vi "Main.vi"(11 "Module Admin":refnum<class "Delacor_lib_QMH_Module Admin.lvclass">) -> ()   [LabVIEW 2021, in "Safety & Release Configuration.lvlib"]
doc: "This template is based off of the Queued Message Handler design pattern and the Queued Message Handler project template that ships with LabVIEW.\n\nThe main difference is that the queue is private to this module and communication between modules is performed via Broadcast and Request events.\n\nRequest events are wrapped in public API methods and are handled in the Event Handling Loop (EHL) of this VI. Any module can register for Broadcast events sent by this module. The EHL generates messages based on user interface actions.\n\nThe Message Handling Loop (MHL) processes messages generated by the EHL, or by other messages. The messages are string values, so new messages can be added easily to the Message Cases case structure in the MHL. Each message cluster can also provide an optional value for Message Data, which is a variant that can be converted to whatever message-specific data is required.\n_____\nBased on DQMH Project Template 7.0.1.1316."
uses:
  Safety & Release Configuration.lvlib
  <vilib>/Delacor/Delacor QMH/Libraries/Module Admin_class/Delacor_lib_QMH_Module Admin.lvclass
  Module Data--cluster.ctl
  Do Something Argument--cluster.ctl
  <vilib>/Delacor/Delacor QMH/Libraries/Message Queue_class/Delacor_lib_QMH_Message Queue.lvclass/Delacor_lib_QMH_Message Queue.ctl
  Do Something Else Argument--cluster.ctl
  Do Something Else and Wait for Reply Argument--cluster.ctl
  Do Something Else and Wait (Reply Payload)--cluster.ctl
  Stop Argument--cluster.ctl
  <vilib>/Delacor/Delacor QMH/Libraries/Module Admin_class/Delacor_lib_QMH_Module Admin.lvclass/Delacor_lib_QMH_Module Admin.ctl
  <vilib>/Utility/miscctls.llb/LVPointTypeDef.ctl
  <vilib>/Delacor/Delacor QMH/Libraries/Message Queue_class/Delacor_lib_QMH_Enqueue Message (Single).vi
  <vilib>/Delacor/Delacor QMH/Libraries/Module Admin_class/Delacor_lib_QMH_Get External Launch.vi
  <vilib>/Delacor/Delacor QMH/Libraries/Message Queue_class/Delacor_lib_QMH_Message Queue.lvclass
  <userlib>/_OpenG.lib/appcontrol/appcontrol.llb/openg_application_control.lvlib
panel:
  in  "Main Tab":enum32{"Release Module", "Safety Module"}(tab)
  in  "Release Module Tab":T1(tab)
  in  "Proximity Sensor 2":u16(ring) items=["Release_Module/port0/line0", "Release_Module/port0/line1", "Release_Module/port0/line2", "Release_Module/port0/line3", "Release_Module/port0/line4", "Release_Module/port0/line5", "Release_Module/port0/line6", "Release_Module/port0/line7", "Release_Module/port0/line8", "Release_Module/port0/line9", "Release_Module/port0/line10", "Release_Module/port0/line11", "Release_Module/port0/line12", "Release_Module/port0/line13", "Release_Module/port0/line14", "Release_Module/port0/line15"]
  in  "Proximity sensor 1":u16(ring) items=["Release_Module/port0/line0", "Release_Module/port0/line1", "Release_Module/port0/line2", "Release_Module/port0/line3", "Release_Module/port0/line4", "Release_Module/port0/line5", "Release_Module/port0/line6", "Release_Module/port0/line7", "Release_Module/port0/line8", "Release_Module/port0/line9", "Release_Module/port0/line10", "Release_Module/port0/line11", "Release_Module/port0/line12", "Release_Module/port0/line13", "Release_Module/port0/line14", "Release_Module/port0/line15"]
  in  "Solenoid Valve":u16(ring) items=["Release_Module/port1/line0", "Release_Module/port1/line1", "Release_Module/port1/line2", "Release_Module/port1/line3", "Release_Module/port1/line4", "Release_Module/port1/line5", "Release_Module/port1/line6", "Release_Module/port1/line7", "Release_Module/port1/line8", "Release_Module/port1/line9", "Release_Module/port1/line10", "Release_Module/port1/line11", "Release_Module/port1/line12", "Release_Module/port1/line13", "Release_Module/port1/line14", "Release_Module/port1/line15"]
  in  "Safety Module Tab":T1(tab)
  in  "Safety Sensor 3":u16(ring) items=["Saftey_Module/port0/line0", "Saftey_Module/port0/line1", "Saftey_Module/port0/line2", "Saftey_Module/port0/line3"]
  in  "Safety Sensor 2":u16(ring) items=["Saftey_Module/port0/line0", "Saftey_Module/port0/line1", "Saftey_Module/port0/line2", "Saftey_Module/port0/line3"]
  in  "Safety Sensor 1":u16(ring) items=["Saftey_Module/port0/line0", "Saftey_Module/port0/line1", "Saftey_Module/port0/line2", "Saftey_Module/port0/line3"]
  in  "Safety Valve 3":u16(ring) items=["Saftey_Module/port0/line4", "Saftey_Module/port0/line5", "Saftey_Module/port0/line6", "Saftey_Module/port0/line7"]
  in  "Safety Valve 2":u16(ring) items=["Saftey_Module/port0/line4", "Saftey_Module/port0/line5", "Saftey_Module/port0/line6", "Saftey_Module/port0/line7"]
  in  "Safety Valve 1":u16(ring) items=["Saftey_Module/port0/line4", "Saftey_Module/port0/line5", "Saftey_Module/port0/line6", "Saftey_Module/port0/line7"]
  in  "Save":bool
  in  "Exit":bool
  out "error out":errorcluster
  out "X":dbl
  out "Status":string
  in  "Simulate MHL Error":bool
  in  "Simulate EHL Error":bool
  in  "Do Something Else <Replace Me>":bool
  in  "Do Something <Replace Me>":bool
  # "IIT-M Drop Tower Test System"
  # "Safety & Release Configuration Window"
  # "These controls have associated \"Value Changed\" events configured in the Event Structure on the diagram.\n\nReplace them (and reconfigure the Event Structure) with the controls you need for your application. \n\nOther processes communicate with this Module via its Public API (wrappers for its Request Events).\n\nThis Module communicates with other processes via its Broadcast Events.\nAny process that wants to receive these messages can register for this module's Broadcast events."
  # "This template is for the DQMH framework. See the block diagram for more information on how to use this template."
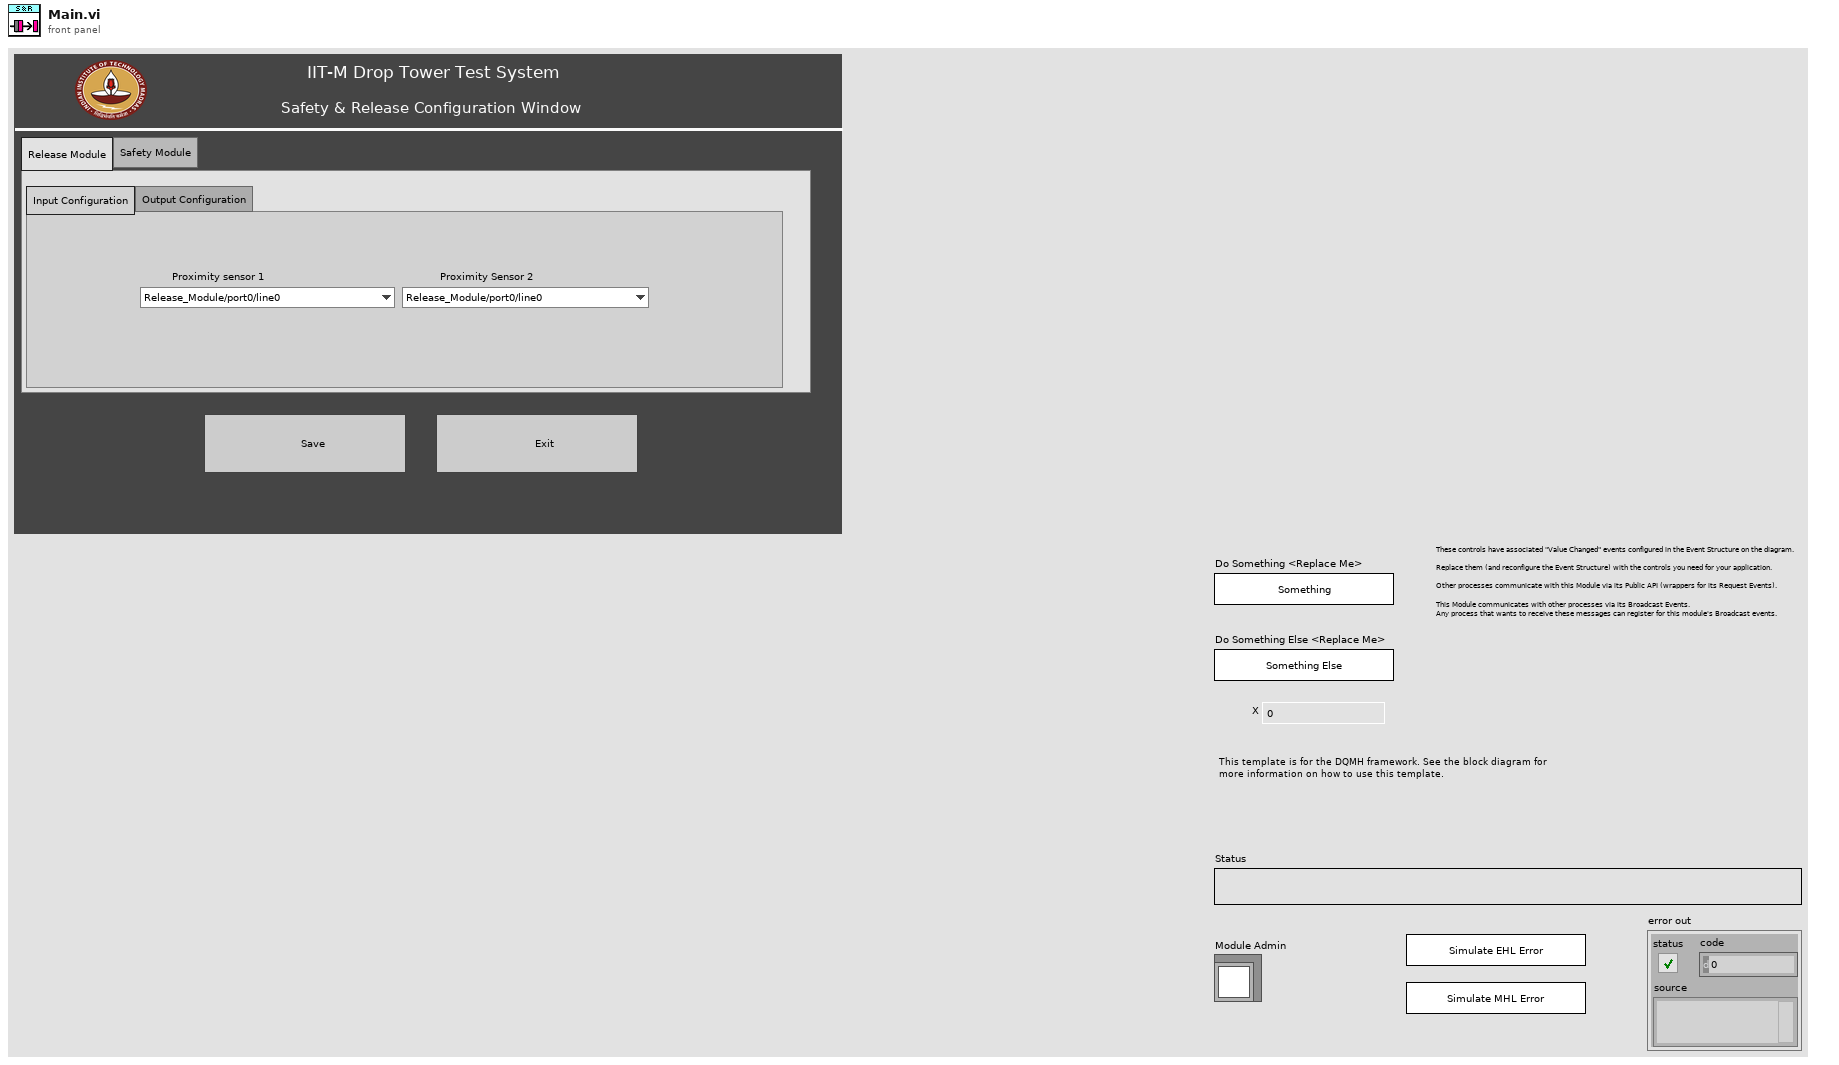
[diagram p1: front panel]
types:
  T1 = enum32{"Input Configuration", "Output Configuration"}
  T2 = typedef "Safety & Release Configuration.lvlib/Request Events--cluster.ctl" = cluster{"Stop Module":refnum<user-event>, "Do Something":refnum<user-event>, "Do Something Else":refnum<user-event>, "Do Something Else and Wait for Reply":refnum<user-event>, "Show Panel":refnum<user-event>, "Hide Panel":refnum<user-event>, "Get Module Execution Status":refnum<user-event>, "Show Diagram":refnum<user-event>}
  T3 = typedef "Safety & Release Configuration.lvlib/Module Data--cluster.ctl" = cluster{"Status":string}
  T4 = typedef "Safety & Release Configuration.lvlib/Do Something Argument--cluster.ctl" = cluster{"Do Something Msg":string}
  T5 = typedef "Safety & Release Configuration.lvlib/Do Something Else Argument--cluster.ctl" = cluster{"Do Something Else Msg":string, "X":dbl}
  T6 = typedef "Safety & Release Configuration.lvlib/Do Something Else and Wait for Reply Argument--cluster.ctl" = cluster{"Do Something Else Msg":string, "X":dbl, "Wait Notifier":refnum<notifier>, "wait for reply":bool}
  T7 = enum32{"invalid lock state", "Not Locked", "Locked (No Password)", "Password-protected"}
  T8 = typedef "Safety & Release Configuration.lvlib/Stop Argument--cluster.ctl" = cluster{"Origin":string, "Exit via Stop Module Req?":bool, "Wait for Module to stop?":bool}
  T9 = typedef "LVPointTypeDef.ctl" = cluster{"Horizontal":i16, "Vertical":i16}
  T10 = enum32{"Invalid", "Standard", "Closed", "Hidden", "Minimized", "Maximized"}
  T11 = typedef "Safety & Release Configuration.lvlib/Do Something Else and Wait (Reply Payload)--cluster.ctl" = cluster{"Value":dbl, "error":errorcluster}
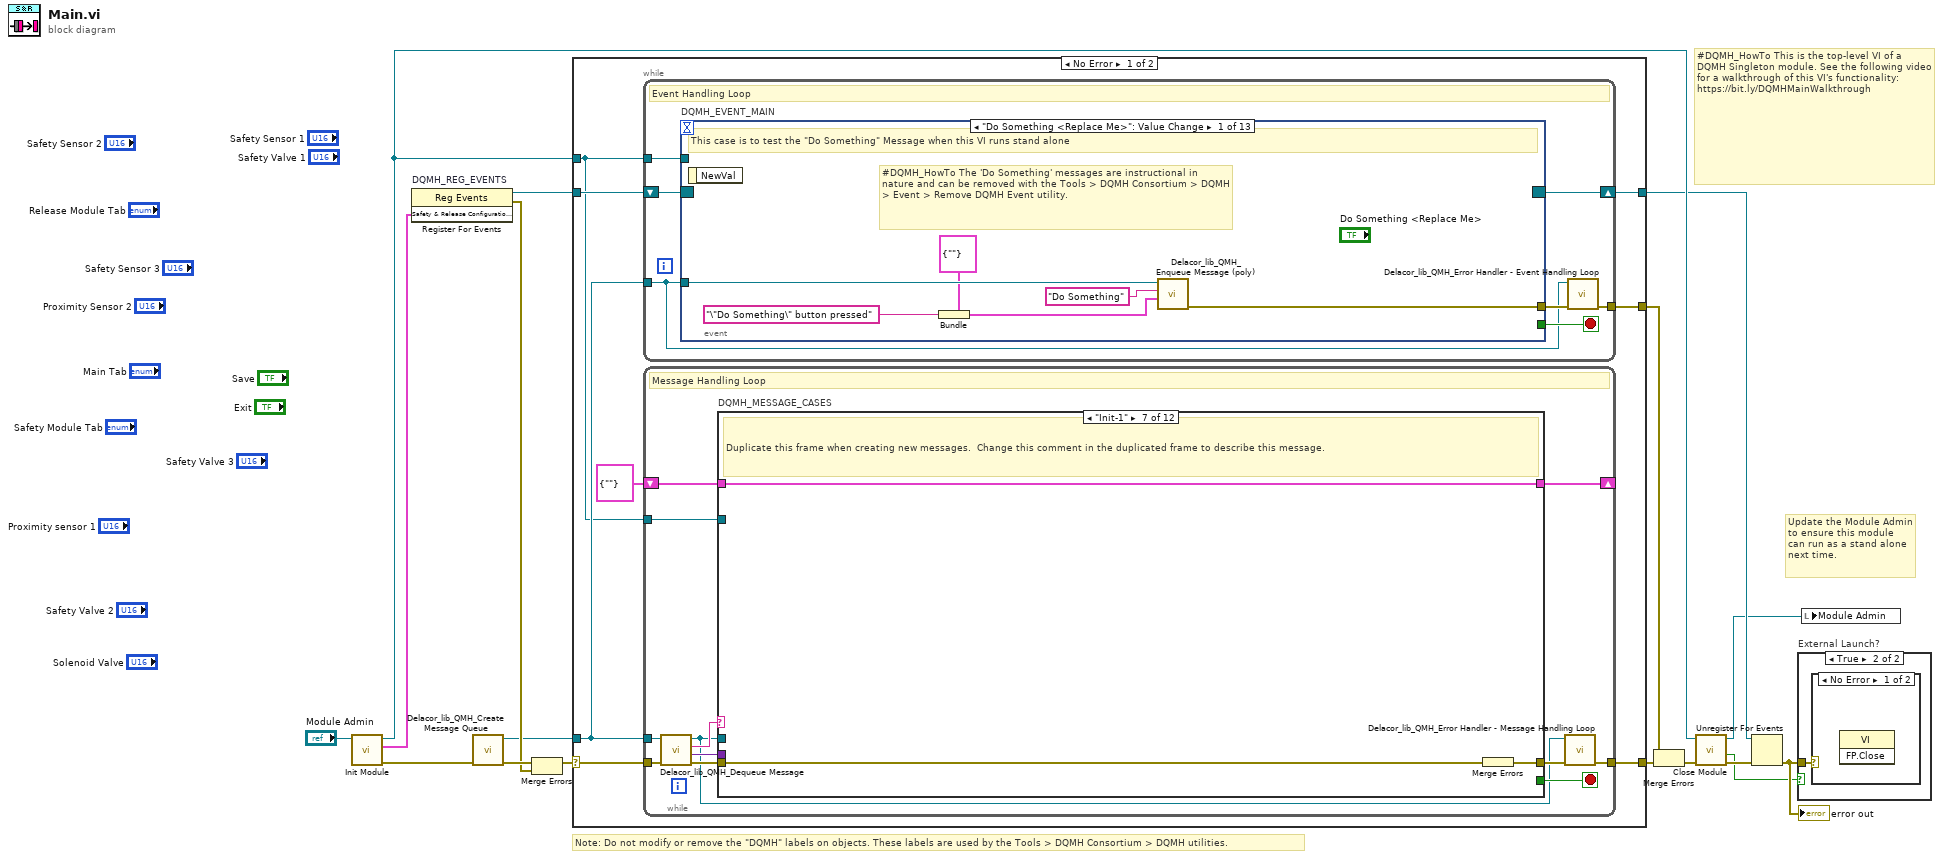
[diagram p0: block diagram]
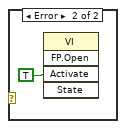
[diagram p3: hidden frame]
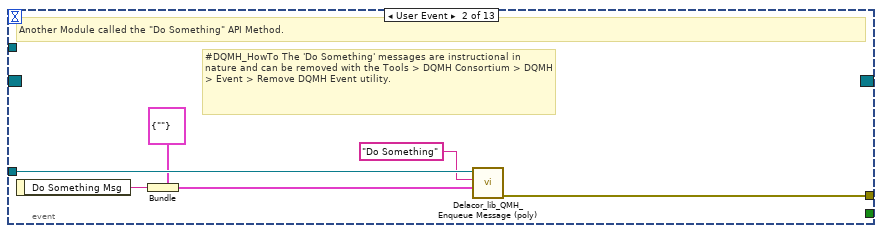
[diagram p4: hidden frame]
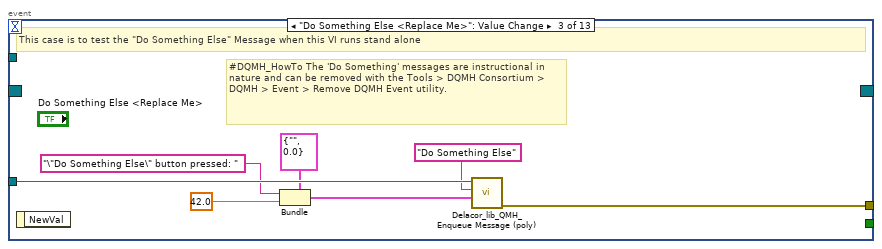
[diagram p5: hidden frame]
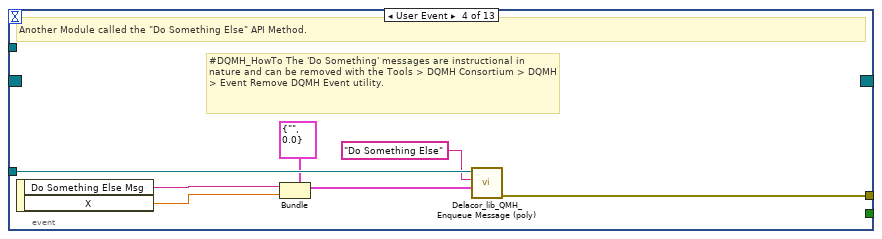
[diagram p6: hidden frame]
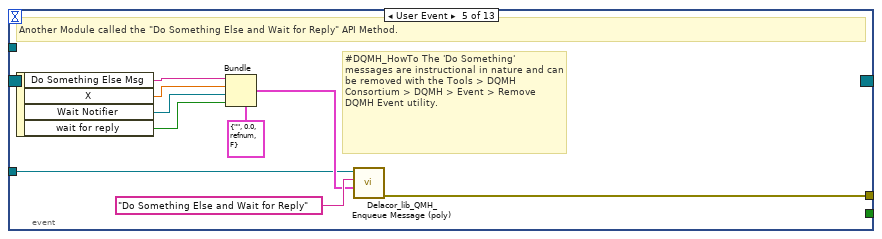
[diagram p7: hidden frame]
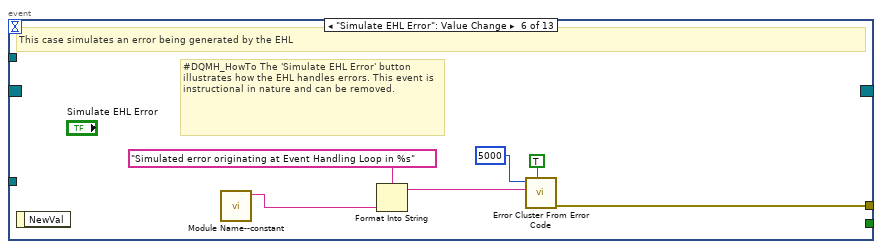
[diagram p8: hidden frame]
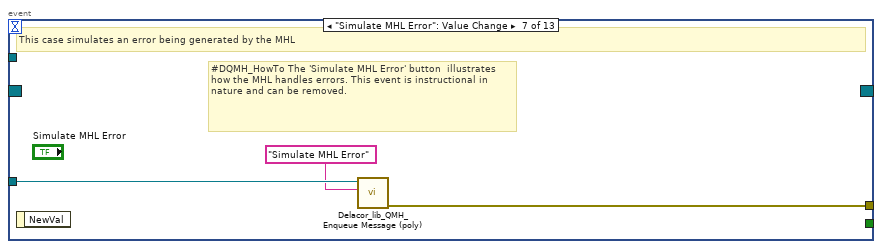
[diagram p9: hidden frame]
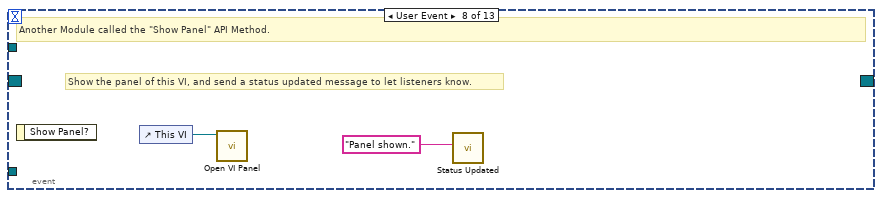
[diagram p10: hidden frame]
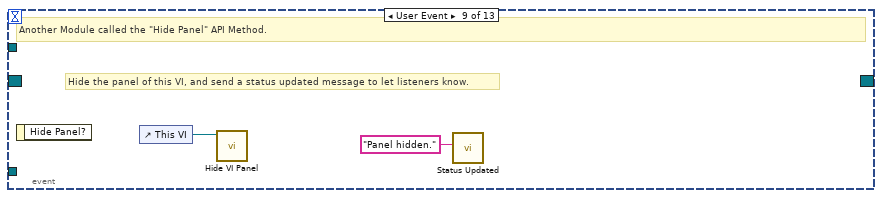
[diagram p11: hidden frame]
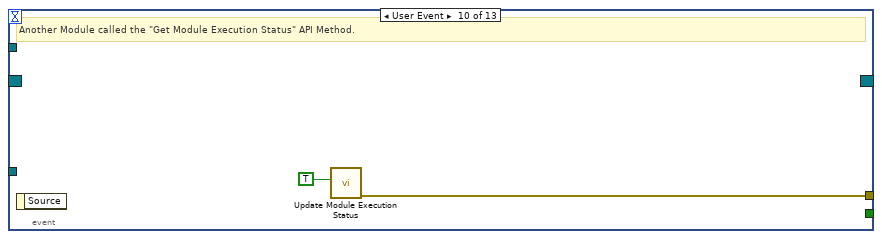
[diagram p12: hidden frame]
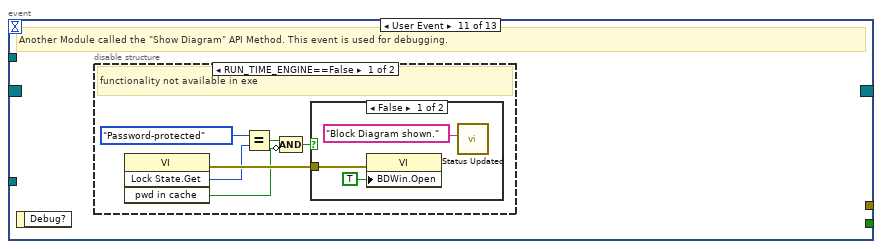
[diagram p13: hidden frame]
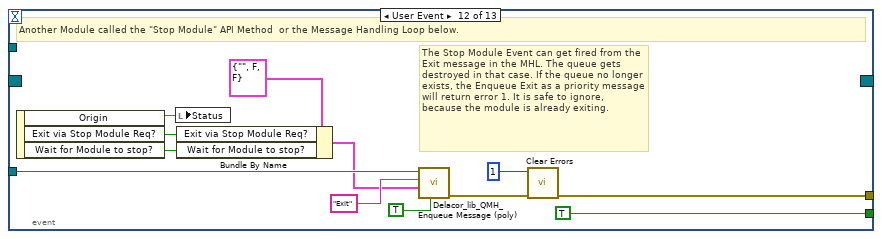
[diagram p16: hidden frame]
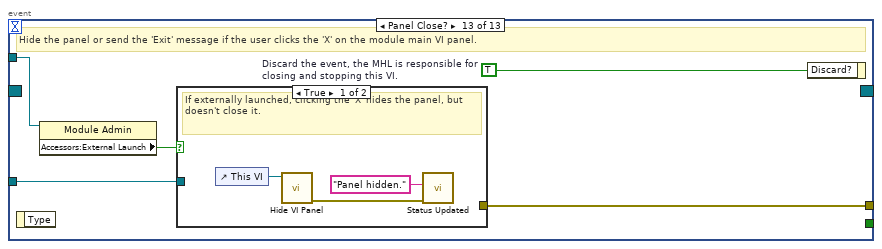
[diagram p17: hidden frame]
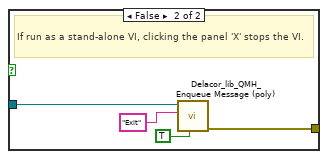
[diagram p18: hidden frame]
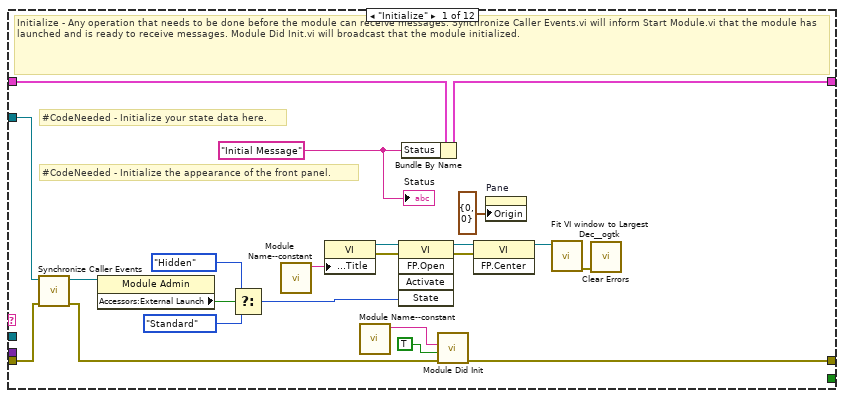
[diagram p19: hidden frame]
diagram:
  # "#DQMH_HowTo This is the top-level VI of a DQMH Singleton module. See the following video for a walkthrough of this VI's functionality: https://bit.ly/DQMHMainWalkthrough"
  # "Note: Do not modify or remove the \"DQMH\" labels on objects. These labels are used by the Tools > DQMH Consortium > DQMH utilities."
  # "Update the Module Admin to ensure this module can run as a stand alone next time."
  n1 = call "Init Module.vi"("Singleton Module Admin in"="Module Admin") -> ("error out"=w16:errorcluster, "Safety & Release Configuration Request Events"=w5:T2, "Singleton Module Admin out"=w8:refnum<class "Delacor_lib_QMH_Module Admin.lvclass">)  [unwired: 8 in]
  n2 = register-events "DQMH_REG_EVENTS"(w5) -> (reference out=w6:refnum<event-registration>, error out=w9:errorcluster)  [unwired: 2 in]
  n3 = call <vilib>:"Delacor_lib_QMH_Create Message Queue.vi"("error in"=w16) -> ("error out"=w11:errorcluster, "Message Queue"=w4:refnum<class "Delacor_lib_QMH_Message Queue.lvclass">)  [unwired: 9 in]
  n4 = Merge Errors(w11, w9) -> (w10:errorcluster)
  n5 = case shown="No Error" w10 {
    selector: w10 -> [w23 w264]
    tunnel: [w25 w263] -> w17
    tunnel: [w22 w262] -> w7
    tunnel: w6 -> [w20 w262]
    tunnel: w4 -> [w19 w257]
    tunnel: [w24 _] -> w14
    tunnel: w8 -> [w18 w258]
    frame No Error {
      n6 = while {
        tunnel: w19 -> [w26]
        shift-right: [w29] -> w22
        shift-left: w20 -> [w30]
        tunnel: [w31] -> w24
        tunnel: w18 -> [w27]
        stop <- w28 stop-if-true
        # "Event Handling Loop"
        n7 = event "DQMH_EVENT_MAIN" shown="[0] \"Do Something <Replace Me>\": Value Change" {
          selector: w30 -> [_ _ _ _ _ _ _ _ _ _ _ _ _]
          dyn-events: [_ _ _ _ _ _ _ _ _ _ _ _ _] -> w29
          timeout: _ -> [_ _ _ _ _ _ _ _ _ _ _ _ _]
          tunnel: [_ _ _ _ _ _ _ _ _ _ _ TRUE ("Discard?") _] -> w28
          tunnel: w26 -> [w37 w43 w50 w57 w60 _ w75 _ _ _ _ w99 w106]
          tunnel: [w38 w44 w51 w58 w67 w73 w76 _ _ w82 _ w102 w108] -> w32
          tunnel: w27 -> [_ _ _ _ _ _ _ _ _ _ _ _ w105]
          event "Do Something <Replace Me>": Value Change {
            # "#DQMH_HowTo The 'Do Something' messages are instructional in nature and can be removed with the Tools > DQMH Consortium > DQMH > Event > Remove DQMH Event utility."
            # "This case is to test the \"Do Something\" Message when this VI runs stand alone"
            n8 = event-data() -> ()  [unwired: 1 in, 1 out]
            n9 = Bundle(cluster=T4 {"Do Something Msg"=""} ("Do Something Argument"), "Do Something Msg"="\"Do Something\" button pressed" ("\"Do Something\" button pressed")) -> (w33:T4)
            n10 = call-poly <vilib>:"Delacor_lib_QMH_Enqueue Message (poly).vi"("Message Data"=w33, "Message"="Do Something", "Message Queue in"=w37) -> ("error out"=w38:errorcluster)  [unwired: 7 in, 1 out]
          }
          event User Event {
            # "#DQMH_HowTo The 'Do Something' messages are instructional in nature and can be removed with the Tools > DQMH Consortium > DQMH > Event > Remove DQMH Event utility."
            # "Another Module called the \"Do Something\" API Method."
            n11 = event-data() -> ("Do Something Msg"=w40:string)  [unwired: 1 in]
            n12 = Bundle(cluster=T4 {"Do Something Msg"=""} ("Do Something Argument"), "Do Something Msg"=w40) -> (w39:T4)
            n13 = call-poly <vilib>:"Delacor_lib_QMH_Enqueue Message (poly).vi"("Message Data"=w39, "Message"="Do Something", "Message Queue in"=w43) -> ("error out"=w44:errorcluster)  [unwired: 7 in, 1 out]
          }
          event "Do Something Else <Replace Me>": Value Change {
            # "#DQMH_HowTo The 'Do Something' messages are instructional in nature and can be removed with the Tools > DQMH Consortium > DQMH > Event > Remove DQMH Event utility."
            # "This case is to test the \"Do Something Else\" Message when this VI runs stand alone"
            n14 = event-data() -> ()  [unwired: 1 in, 1 out]
            n15 = Bundle(cluster=T5 {"Do Something Else Msg"="", "X"=0.0} ("Do Something Else Argument"), "Do Something Else Msg"="\"Do Something Else\" button pressed: " ("\"Do Something Else\" button pressed"), "X"=42.0) -> (w47:T5)
            n16 = call-poly <vilib>:"Delacor_lib_QMH_Enqueue Message (poly).vi"("Message Data"=w47, "Message"="Do Something Else", "Message Queue in"=w50) -> ("error out"=w51:errorcluster)  [unwired: 7 in, 1 out]
          }
          event User Event {
            # "#DQMH_HowTo The 'Do Something' messages are instructional in nature and can be removed with the Tools > DQMH Consortium > DQMH > Event Remove DQMH Event utility."
            # "Another Module called the \"Do Something Else\" API Method."
            n17 = event-data() -> ("Do Something Else Msg"=w53:string, "X"=w52:dbl)  [unwired: 1 in]
            n18 = Bundle(cluster=T5 {"Do Something Else Msg"="", "X"=0.0} ("Do Something Else Argument"), "Do Something Else Msg"=w53, "X"=w52) -> (w54:T5)
            n19 = call-poly <vilib>:"Delacor_lib_QMH_Enqueue Message (poly).vi"("Message Data"=w54, "Message"="Do Something Else", "Message Queue in"=w57) -> ("error out"=w58:errorcluster)  [unwired: 7 in, 1 out]
          }
          event User Event {
            # "#DQMH_HowTo The 'Do Something' messages are instructional in nature and can be removed with the Tools > DQMH Consortium > DQMH > Event > Remove DQMH Event utility."
            # "Another Module called the \"Do Something Else and Wait for Reply\" API Method."
            n20 = event-data() -> ("Do Something Else Msg"=w63:string, "X"=w62:dbl, "Wait Notifier"=w61:refnum<notifier>, "wait for reply"=w59:bool)  [unwired: 1 in]
            n21 = Bundle(cluster=T6 {"Do Something Else Msg"="", "X"=0.0, "Wait Notifier"=refnum, "wait for reply"=FALSE} ("Do Something Else and Wait for Reply Argument"), "Do Something Else Msg"=w63, "X"=w62, "Wait Notifier"=w61, "wait for reply"=w59) -> (w64:T6)
            n22 = call-poly <vilib>:"Delacor_lib_QMH_Enqueue Message (poly).vi"("Message Data"=w64, "Message"="Do Something Else and Wait for Reply", "Message Queue in"=w60) -> ("error out"=w67:errorcluster)  [unwired: 7 in, 1 out]
          }
          event "Simulate EHL Error": Value Change {
            # "#DQMH_HowTo The 'Simulate EHL Error' button  illustrates how the EHL handles errors. This event is instructional in nature and can be removed."
            # "This case simulates an error being generated by the EHL"
            n23 = event-data() -> ()  [unwired: 1 in, 1 out]
            n24 = call "Module Name--constant.vi"() -> ("Module Name"=w70:string)  [unwired: 11 in]
            n25 = Format Into String(format string="Simulated error originating at Event Handling Loop in %s", w70) -> (resulting string=w71:string)  [unwired: 2 in, 1 out]
            n26 = call <vilib>:"Error Cluster From Error Code.vi"("show call chain? (False)"=TRUE, "error message (\"\")"=w71, "error code (0)"=5000) -> ("error out"=w73:errorcluster)  [unwired: 6 in]
          }
          event "Simulate MHL Error": Value Change {
            # "#DQMH_HowTo The 'Simulate MHL Error' button  illustrates how the MHL handles errors. This event is instructional in nature and can be removed."
            # "This case simulates an error being generated by the MHL"
            n27 = event-data() -> ()  [unwired: 1 in, 1 out]
            n28 = call-poly <vilib>:"Delacor_lib_QMH_Enqueue Message (poly).vi"("Message"="Simulate MHL Error", "Message Queue in"=w75) -> ("error out"=w76:errorcluster)  [unwired: 8 in, 1 out]
          }
          event User Event {
            # "Show the panel of this VI, and send a status updated message to let listeners know."
            # "Another Module called the \"Show Panel\" API Method."
            n29 = event-data() -> ()  [unwired: 1 in, 1 out]
            n30 = control-ref of="This VI"() -> (w78:refnum<vi>)
            n31 = call "Open VI Panel.vi"("VI"=w78) -> ()  [unwired: 10 in, 1 out]
            n32 = call "Status Updated.vi"("Status"="Panel shown." ("format string")) -> ()  [unwired: 10 in, 1 out]
          }
          event User Event {
            # "Hide the panel of this VI, and send a status updated message to let listeners know."
            # "Another Module called the \"Hide Panel\" API Method."
            n33 = event-data() -> ()  [unwired: 1 in, 1 out]
            n34 = control-ref of="This VI"() -> (w80:refnum<vi>)
            n35 = call "Hide VI Panel.vi"("VI"=w80) -> ()  [unwired: 10 in, 1 out]
            n36 = call "Status Updated.vi"("Status"="Panel hidden." ("format string")) -> ()  [unwired: 10 in, 1 out]
          }
          event User Event {
            # "Another Module called the \"Get Module Execution Status\" API Method."
            n37 = event-data() -> ()  [unwired: 1 in, 1 out]
            n38 = call "Update Module Execution Status.vi"("Running?"=TRUE) -> ("error out"=w82:errorcluster)  [unwired: 10 in]
          }
          event User Event {
            # "Another Module called the \"Show Diagram\" API Method. This event is used for debugging."
            n39 = event-data() -> ()  [unwired: 1 in, 1 out]
            n40 = disable-structure shown="RUN_TIME_ENGINE==False" {
              frame condition #0 (active) {
                # "functionality not available in exe"
                n41 = invoke on="Invoke Node" class="VI" method="Lock State.Get"() -> (error out=w88:errorcluster, "Get Lock State"=w87:T7, "pwd in cache"=w84:bool)  [unwired: 4 in, 1 out]
                n42 = Equal?(x=T7."Password-protected", y=w87) -> (x = y?=w85:bool)
                n43 = Compound Arithmetic op=AND(w85, invert w84) -> (w83:bool)
                n44 = case shown="False" w83 {
                  tunnel: w88 -> [w91 _]
                  frame False {
                    n45 = property on="Property Node" class="VI"(error in=w91, "BDWin.Open"=TRUE ("Block Diagram Window:Open")) -> ()  [unwired: 1 in, 2 out]
                    n46 = call "Status Updated.vi"("Status"="Block Diagram shown." ("format string")) -> ()  [unwired: 10 in, 1 out]
                  }
                  frame True {
                    # "Password-protected VI, and the password is not in the cache. Do not show the diagram."
                  }
                }
              }
              frame condition #1 {
              }
            }
          }
          event User Event {
            # "The Stop Module Event can get fired from the Exit message in the MHL. The queue gets destroyed in that case. If the queue no longer exists, the Enqueue Exit as a priority message will return error 1. It is safe to ignore, because the module is already exiting."
            # "Another Module called the \"Stop Module\" API Method  or the Message Handling Loop below."
            n47 = event-data() -> ("Origin"=w98:string, "Exit via Stop Module Req?"=w94:bool, "Wait for Module to stop?"=w93:bool)  [unwired: 1 in]
            n48 = local write "Status"(w98) -> ()
            n49 = Bundle By Name(cluster=T8 {"Origin"="", "Exit via Stop Module Req?"=FALSE, "Wait for Module to stop?"=FALSE} ("Stop Argument"), "Exit via Stop Module Req?"=w94, "Wait for Module to stop?"=w93) -> (w92:T8)
            n50 = call-poly <vilib>:"Delacor_lib_QMH_Enqueue Message (poly).vi"("Priority Message? (F)"=TRUE, "Message Data"=w92, "Message"="Exit", "Message Queue in"=w99) -> ("error out"=w103:errorcluster)  [unwired: 6 in, 1 out]
            n51 = call <vilib>:"Clear Errors.vi"("error in (no error)"=w103, "specific error code to clear (0: all)"=1) -> ("error out"=w102:errorcluster)  [unwired: 4 in, 1 out]
          }
          event Panel Close? {
            w107 = TRUE  # Discard the event, the MHL is responsible for closing and stopping this VI.
            # "Hide the panel or send the 'Exit' message if the user clicks the 'X' on the module main VI panel."
            n52 = event-data() -> ()  [unwired: 1 in, 1 out]
            n53 = property on="Property Node" class="Module Admin"(reference=w105) -> ("Accessors:External Launch"=w104:bool)  [unwired: 1 in, 2 out]
            n54 = case shown="True" w104 {
              tunnel: w106 -> [_ w114]
              tunnel: [_ w115] -> w108
              frame True {
                # "If externally launched, clicking the 'X' hides the panel, but doesn't close it."
                n55 = control-ref of="This VI"() -> (w111:refnum<vi>)
                n56 = call "Hide VI Panel.vi"("VI"=w111) -> ("error out"=w109:errorcluster)  [unwired: 10 in]
                n57 = call "Status Updated.vi"("error in"=w109, "Status"="Panel hidden." ("format string")) -> ()  [unwired: 9 in, 1 out]
              }
              frame False {
                # "If run as a stand-alone VI, clicking the panel 'X' stops the VI."
                n58 = call-poly <vilib>:"Delacor_lib_QMH_Enqueue Message (poly).vi"("Priority Message? (F)"=TRUE, "Message"="Exit", "Message Queue in"=w114) -> ("error out"=w115:errorcluster)  [unwired: 7 in, 1 out]
              }
            }
            n59 = event-data ("Event Filter Node")("Discard?"=w107) -> ()  [unwired: 1 in, 1 out]
          }
        }
        n60 = call-dynamic "Delacor_lib_QMH_Error Handler - Event Handling Loop.vi"("error in"=w32, "Message Queue in"=w26) -> ("dup error in"=w31:errorcluster)  [unwired: 8 in, 1 out]
      }
      n61 = while {
        tunnel: w19 -> [w116]
        shift-right: [w124] -> _
        shift-left: T3 {"Status"=""} ("Data Cluster") -> [w125]
        tunnel: w23 -> [w127]
        tunnel: [w119] -> w25
        tunnel: w18 -> [w120]
        stop <- w123 stop-if-true
        # "Message Handling Loop"
        n62 = call-dynamic "Delacor_lib_QMH_Dequeue Message.vi"("error in"=w127, "Message Queue in"=w116) -> ("error out"=w126:errorcluster, "Message Data"=w121:variant, "Message"=w122:string, "Message Queue out"=w117:refnum<class "Delacor_lib_QMH_Message Queue.lvclass">)  [unwired: 6 in]
        n63 = case "DQMH_MESSAGE_CASES" shown="\"Init-1\"" w122 {
          selector: w122 -> [_ _ _ _ _ _ _ _ _ _ _ w252]
          tunnel: w117 -> [_ _ _ _ _ _ _ _ _ w218 w240 _]
          tunnel: w126 -> [w147 w151 w159 w168 w187 w200 w203 w205 w214 w225 w246 w255]
          tunnel: [w145 w151 w157 w167 w186 w199 w202 w205 w213 w221 w241 w256] -> w118
          tunnel: w125 -> [w136 w150 w156 w166 w183 w198 w201 w204 w211 w220 w239 w253]
          tunnel: [w135 w150 w156 w166 w183 w198 w201 w204 w211 w220 w239 w253] -> w124
          tunnel: [_ _ _ _ _ _ _ _ _ _ w238 _] -> w123
          tunnel: w121 -> [_ _ w155 w163 w180 _ _ _ _ w219 w237 _]
          tunnel: w120 -> [w137 _ _ _ _ _ _ _ _ w217 w232 _]
          frame "Initialize" {
            w131 = "Initial Message" ("Initial Message")
            # "#CodeNeeded - Initialize the appearance of the front panel."
            # "#CodeNeeded - Initialize your state data here."
            # "Initialize - Any operation that needs to be done before the module can receive messages. Synchronize Caller Events.vi will inform Start Module.vi that the module has launched and is ready to receive messages. Module Did Init.vi will broadcast that the module initialized."
            n64 = call "Synchronize Caller Events.vi"("error in"=w147, "Singleton Module Admin in"=w137) -> ("error out"=w146:errorcluster, "Singleton Module Admin out"=w132:refnum<class "Delacor_lib_QMH_Module Admin.lvclass">)  [unwired: 8 in]
            n65 = property on="Property Node" class="Module Admin"(reference=w132) -> ("Accessors:External Launch"=w141:bool)  [unwired: 1 in, 2 out]
            n66 = Select(t=T10."Hidden" ("State"), s=w141, f=T10."Standard" ("State")) -> (s? t:f=w138:T10)
            n67 = call "Module Name--constant.vi"() -> ("Module Name"=w144:string)  [unwired: 11 in]
            n68 = property on="Property Node" class="VI"("Front Panel.Title"=w144) -> (reference out=w143:refnum<vi>, error out=w149:errorcluster)  [unwired: 2 in]
            n69 = call "Module Name--constant.vi"() -> ("Module Name"=w133:string)  [unwired: 11 in]
            n70 = invoke on="Invoke Node" class="VI" method="FP.Open"(reference=w143, error in=w149, "State"=w138) -> (reference out=w142:refnum<vi>, error out=w148:errorcluster)  [unwired: 2 in, 3 out]
            n71 = Bundle By Name(cluster=w136, "Status"=w131) -> (w135:T3)
            n72 = call "Module Did Init.vi"("error in"=w146, "Initialized?"=TRUE, "Origin"=w133) -> ("error out"=w145:errorcluster)  [unwired: 8 in]
            n73 = invoke on="Invoke Node" class="VI" method="FP.Center"(reference=w142, error in=w148) -> (reference out=w129:refnum<vi>)  [unwired: 1 in, 2 out]
            n74 = property on="Pane" class="Pane"("Origin"=T9 {"Horizontal"=0, "Vertical"=0}) -> ()  [unwired: 2 in, 2 out]
            n75 = call <userlib>:"Fit VI window to Largest Dec__ogtk.vi"("VI Ref (calling VI)"=w129) -> ("error out"=w128:errorcluster)  [unwired: 5 in, 1 out]
            n76 = call <vilib>:"Clear Errors.vi"("error in (no error)"=w128) -> ()  [unwired: 5 in, 2 out]
            "Status" <- w131
          }
          frame "---Module Specific---" {
            # "Separator -- The following cases handle messages specific to this Module."
          }
          frame "Do Something" {
            # "#DQMH_HowTo The 'Do Something' messages are instructional in nature and can be removed with the Tools > DQMH Consortium > DQMH > Event > Remove DQMH Event utility."
            # "Do Something - Replace this message with functionality for your own application. Note that this message also fires the \"Did Something\" broadcast event."
            n77 = Variant To Data(error in=w159, type=T4 {"Do Something Msg"=""} ("Do Something Argument"), Variant=w155) -> (data=w154:T4, error out=w158:errorcluster)
            n78 = Unbundle By Name(w154) -> ("Do Something Msg"=w152:string)
            n79 = call "Did Something.vi"("error in"=w158, "Did Something Msg"=w152) -> ("error out"=w157:errorcluster)  [unwired: 9 in]
            n80 = local write "Status"(w152) -> ()
            n81 = call "Status Updated.vi"("Status"=w152) -> ()  [unwired: 10 in, 1 out]
          }
          frame "Do Something Else" {
            # "#DQMH_HowTo The 'Do Something' messages are instructional in nature and can be removed with the Tools > DQMH Consortium > DQMH > Event > Remove DQMH Event utility."
            # "Do Something Else - Replace this message with functionality for your own application."
            n82 = Variant To Data(error in=w168, type=T5 {"Do Something Else Msg"="", "X"=0.0} ("Do Something Else Argument"), Variant=w163) -> (data=w164:T5, error out=w167:errorcluster)
            n83 = Unbundle By Name(w164) -> ("Do Something Else Msg"=w162:string, "X"=w161:dbl)
            "X" <- w161
            n84 = Format Into String(initial string=w162, w161) -> (resulting string=w160:string)  [unwired: 2 in, 1 out]
            n85 = local write "Status"(w160) -> ()
            n86 = call "Status Updated.vi"("Status"=w160) -> ()  [unwired: 10 in, 1 out]
          }
          frame "Do Something Else and Wait for Reply" {
            w175 = "X(%.2f)+Offset(%.2f)=%.2f"  # status message format string
            # "#DQMH_HowTo The 'Do Something' messages are instructional in nature and can be removed."
            # "Send back X with a random offset"
            # "Do Something Else and Wait for Reply - Replace this message with functionality for your own application. Note that this message must fire a notifier to let callers know it has finished execution, and it returns an error if the 'Value' is negative."
            n87 = Variant To Data(error in=w187, type=T6 {"Do Something Else Msg"="", "X"=0.0, "Wait Notifier"=refnum, "wait for reply"=FALSE} ("Do Something Else and Wait for Reply Argument"), Variant=w180) -> (data=w181:T6, error out=w185:errorcluster)
            n88 = Unbundle By Name(w181) -> ("Wait Notifier"=w169:refnum<notifier>, "Do Something Else Msg"=w179:string, "X"=w176:dbl, "wait for reply"=w172:bool)
            n89 = Random Number (0-1)() -> (number: 0 to 1=w177:dbl)
            n90 = Add(x=w177, y=w176) -> (x+y=w171:dbl)
            n91 = Less Than 0?(x=w171) -> (x < 0?=w174:bool)
            n92 = local write "X"(w176) -> ()
            n93 = case shown="True" w174 {
              tunnel: [_ w197] -> w184
              frame False {
              }
              frame True {
                n94 = call <vilib>:"Error Cluster From Error Code.vi"("show call chain? (False)"=TRUE, "error message (\"\")"="The 'Something Else and Wait for Reply' message generated a negative number, which is considered an error condition.", "error code (0)"=5000) -> ("error out"=w197:errorcluster)  [unwired: 6 in]
              }
            }
            n95 = Format Into String(format string=w175, initial string=w179, w176, w177, w171) -> (resulting string=w173:string)  [unwired: 1 in, 1 out]
            n96 = Bundle By Name(cluster=T11 {"Value"=0.0, "error"={"status"=FALSE, "code"=0, "source"=""}} ("notification"), "error"=w184, "Value"=w171) -> (w170:T11)
            n97 = local write "Status"(w173) -> ()
            n98 = call "Status Updated.vi"("Status"=w173) -> ()  [unwired: 10 in, 1 out]
            n99 = case shown="True" w172 {
              tunnel: w170 -> [_ w190]
              tunnel: w169 -> [_ w189]
              frame False {
              }
              frame True {
                # "Simulate an operation that requires a wait."
                n100 = flat-sequence {
                  tunnel: w190 -> [w193]
                  tunnel: w189 -> [w192]
                  tunnel: w188 -> [_]
                  frame #0 {
                    n101 = Send Notification(notification=w193, notifier=w192) -> ()  [unwired: 1 in, 2 out]
                  }
                }
                n102 = Wait (ms)(milliseconds to wait=u32 1000) -> (millisecond timer value=w188:u32)
              }
            }
            n103 = Merge Errors(w185, w184) -> (w186:errorcluster)
          }
          frame "---Copy This Frame---" {
            # "Duplicate this frame when creating new messages.  Change this comment in the duplicated frame to describe this message."
            n104 = Merge Errors(w200) -> (w199:errorcluster)
          }
          frame "Init-1" {
            # "Duplicate this frame when creating new messages.  Change this comment in the duplicated frame to describe this message."
            n105 = Merge Errors(w203) -> (w202:errorcluster)
          }
          frame "---Exit and Error Handling---" {
            # "Separator - The following cases handle errors and exit messages."
          }
          frame "Simulate MHL Error" {
            # "#DQMH_HowTo The 'Simulate MHL Error' button  illustrates how the MHL handles errors. This event is instructional in nature and can be removed."
            # "Simulate an error occurring at the MHL"
            n106 = call "Module Name--constant.vi"() -> ("Module Name"=w207:string)  [unwired: 11 in]
            n107 = Format Into String(format string="Simulated error originating at Message Handling Loop in %s", w207) -> (resulting string=w208:string)  [unwired: 2 in, 1 out]
            n108 = call <vilib>:"Error Cluster From Error Code.vi"("show call chain? (False)"=TRUE, "error message (\"\")"=w208, "error code (0)"=5001) -> ("error out"=w212:errorcluster)  [unwired: 6 in]
            n109 = Merge Errors(w214, w212) -> (w213:errorcluster)
          }
          frame "Error" {
            # "#CodeRecommended - If the module is running in standalone mode (External Launch = FALSE), this code will pop up an error dialog and call the 'Exit' message if an error occurs. Add more fine-grained error management here."
            # "Error - Check the error message data and respond accordingly. This message is sent by the \"Error Handler\" VIs at the end of each loop in this application."
            n110 = property on="Property Node" class="Module Admin"(reference=w217) -> ("Accessors:External Launch"=w216:bool)  [unwired: 1 in, 2 out]
            n111 = Variant To Data(error in=w225, type=errorcluster {"status"=FALSE, "code"=0, "source"=""} ("error constant"), Variant=w219) -> (data=w215:errorcluster, error out=w223:errorcluster)
            n112 = local write "error out"(w215) -> ()
            n113 = call "Error Reported.vi"("Error"=w215) -> ()  [unwired: 10 in, 1 out]
            n114 = case shown="False" w216 {
              tunnel: [w230 _] -> w222
              tunnel: w218 -> [w228 _]
              tunnel: w215 -> [w229 _]
              frame False {
                n115 = disable-structure shown="Default" {
                  disable-tunnel: w229 -> [w231 _]
                  frame condition #0 (active) {
                    # "If the module is running standalone, then pop up an error dialog and call the \"Exit\" message."
                    n116 = call <vilib>:"Simple Error Handler.vi"("error in (no error)"=w231) -> ()  [unwired: 4 in, 5 out]
                  }
                  frame condition #1 {
                    # "To prevent the Simple Error Handler VI from being loaded (e.g. when deploying to a Real-Time target), add the Conditional Disable Symbol \"DQMH_Disable_SEH\" to your project and set it to TRUE."
                  }
                }
                n117 = call-poly <vilib>:"Delacor_lib_QMH_Enqueue Message (poly).vi"("Priority Message? (F)"=TRUE, "Message"="Exit", "Message Queue in"=w228) -> ("error out"=w230:errorcluster)  [unwired: 7 in, 1 out]
              }
              frame True {
                # "If the module was launched externally, calling the Error Reported broadcast VI is the only action performed by the \"Error\" message. The module's caller can then process the error appropriately."
              }
            }
            n118 = Merge Errors(w223, w222) -> (w221:errorcluster)
          }
          frame "Exit" {
            w236 = 91  # 91: not all Exit messages will have an argument
            w238 = TRUE  # Stop the VI
            # "Release the message queue reference"
            # "#CodeNeeded - Add any required cleanup code here."
            # "Exit - Exit the application."
            n119 = Variant To Data(error in=w246, type=T8 {"Origin"="", "Exit via Stop Module Req?"=FALSE, "Wait for Module to stop?"=FALSE} ("Stop Argument"), Variant=w237) -> (data=w234:T8, error out=w243:errorcluster)
            n120 = call <vilib>:"Clear Errors.vi"("error in (no error)"=w243, "specific error code to clear (0: all)"=w236) -> ("error out"=w245:errorcluster)  [unwired: 4 in, 1 out]
            n121 = control-ref of="This VI"() -> (w233:refnum<vi>)
            n122 = call-dynamic "Delacor_lib_QMH_Release Message Queue.vi"("error in"=w245, "Message Queue"=w240) -> ("error out"=w244:errorcluster)  [unwired: 9 in]
            n123 = call "Handle Exit.vi"("Stop Argument"=w234, "Admin in"=w232, "VI reference"=w233) -> ("error out"=w242:errorcluster)  [unwired: 7 in, 1 out]
            n124 = Merge Errors(w244, w242) -> (w241:errorcluster)
            n125 = call "Error Reported.vi"("Error"=w241) -> ()  [unwired: 10 in, 1 out]
          }
          frame Default {
            # "'Default' case only runs if there is a message that isn't defined in any of the other cases.  Output a programming error."
            n126 = call "Module Name--constant.vi"() -> ("Module Name"=w251:string)  [unwired: 11 in]
            n127 = Format Into String(format string="The invalid message string \"%s\" was received in the Message Handling Loop for module \"%s\".", w252, w251) -> (resulting string=w247:string)  [unwired: 2 in, 1 out]
            n128 = call <vilib>:"Error Cluster From Error Code.vi"("show call chain? (False)"=TRUE, "error message (\"\")"=w247, "error code (0)"=1) -> ("error out"=w254:errorcluster)  [unwired: 6 in]
            n129 = Merge Errors(w255, w254) -> (w256:errorcluster)
          }
        }
        n130 = call-dynamic "Delacor_lib_QMH_Error Handler - Message Handling Loop.vi"("error in"=w118, "Message Queue in"=w117) -> ("dup error in"=w119:errorcluster)  [unwired: 8 in, 1 out]
      }
    }
    frame Error {
      # "Synchronize Caller Events.vi will inform Start Module.vi that the module has launched and will let the code calling Start Module.vi register for broadcasts and would permit the caller receive the broadcast that an error occurred at launch time."
      n131 = call-dynamic "Delacor_lib_QMH_Release Message Queue.vi"("error in"=w264, "Message Queue"=w257) -> ("error out"=w263:errorcluster)  [unwired: 9 in]
      n132 = call "Synchronize Caller Events.vi"("Singleton Module Admin in"=w258) -> ("error out"=w265:errorcluster)  [unwired: 9 in, 1 out]
      n133 = call "Module Name--constant.vi"() -> ("Module Name"=w261:string)  [unwired: 11 in]
      n134 = Format Into String(format string="An error occurred during initialization. %s is no longer running.", w261) -> (resulting string=w259:string)  [unwired: 2 in, 1 out]
      n135 = Merge Errors(w263, w265) -> (w266:errorcluster)
      n136 = call "Error Reported.vi"("Additional Information"=w259, "Error"=w266) -> ()  [unwired: 9 in, 1 out]
    }
  }
  n137 = Merge Errors(w14, w17) -> (w13:errorcluster)
  n138 = call "Close Module.vi"("error in"=w13, "Module Admin in"=w8) -> ("error out"=w15:errorcluster, "External Launch"=w1:bool, "Module Admin out"=w2:refnum<class "Delacor_lib_QMH_Module Admin.lvclass">)  [unwired: 7 in]
  n139 = Unregister For Events(event registration refnum=w7, error in=w15) -> (error out=w12:errorcluster)
  "error out" <- w12
  n140 = case "External Launch?" shown="True" w1 {
    tunnel: w12 -> [_ w267]
    frame False {
    }
    frame True {
      n141 = case shown="No Error" w267 {
        frame No Error {
          n142 = invoke on="Invoke Node" class="VI" method="FP.Close"() -> ()  [unwired: 3 in, 3 out]
        }
        frame Error {
          n143 = invoke on="Invoke Node" class="VI" method="FP.Open"("Activate"=TRUE ("Activate?")) -> ()  [unwired: 4 in, 5 out]
        }
      }
    }
  }
  n144 = local write "Module Admin"(w2) -> ()
